vi "From PDM task.vi"(10 "PDM input task":refnum<data-value>) -> (2 "task":u64)   [LabVIEW 2022 SP3, in "DAAG task conversion.lvlib"]
uses:
  DAAG task conversion.lvlib
  <vilib>/PDM Acquisition Toolkit/host/Classes/Tasks/PDM Tasks/PDM Task.lvclass
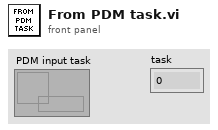
[diagram p1: front panel]
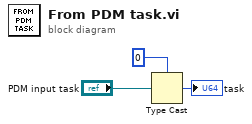
[diagram p0: block diagram]
diagram:
  n1 = Type Cast(type=u64 0, x="PDM input task") -> (*(type *) &x=→"task":u64)
